vi "MT Generate PSK Symbol Map.vi"(0 "symbol values":i32[](array[numeric]), 11 "error in (no error)":errorcluster) -> (4 "symbol map":cdb[](array[numeric]) format="%.3f", 6 "bits per symbol":i32, 15 "error out":errorcluster)   [LabVIEW 2020, in "niDMT.lvlib"]
uses:
  <vilib>/addons/Modulation/niDMT.lvlib
  <vilib>/addons/Modulation/niAMT.lvlib
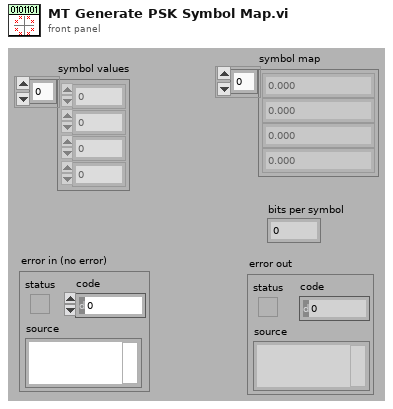
[diagram p1: front panel]
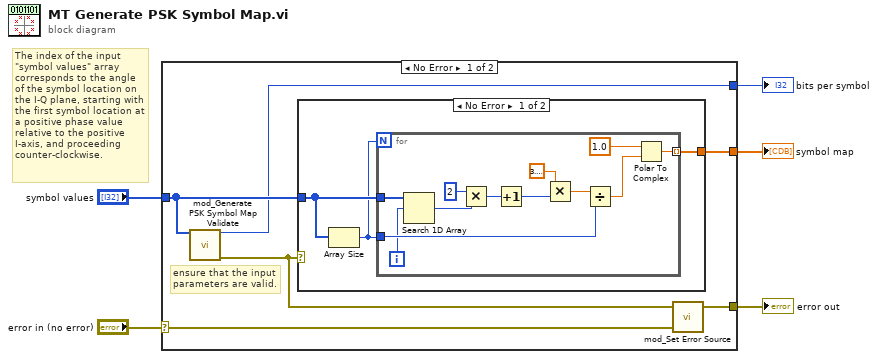
[diagram p0: block diagram]
diagram:
  # "The index of the input \"symbol values\" array corresponds to the angle of the symbol location on the I-Q plane, starting with the first symbol location at a positive phase value relative to the positive I-axis, and proceeding counter-clockwise."
  n1 = case shown="No Error" "error in (no error)" {
    selector: "error in (no error)" -> [w11 w27]
    tunnel: "symbol values" -> [w9 _]
    tunnel: [w10 w27] -> w4
    tunnel: [w8 _] -> w2
    tunnel: [w6 _] -> w1
    frame No Error {
      # "ensure that the input parameters are valid."
      n2 = call <vilib>:"mod_Generate PSK Symbol Map Validate.vi"("Symbol Map"=w9) -> ("bits per symbol"=w6:i32, "error out"=w7:errorcluster)  [unwired: 13 out]
      n3 = case shown="No Error" w7 {
        tunnel: w9 -> [w14 _]
        tunnel: [w13 _] -> w8
        frame No Error {
          n4 = Array Size(array=w14) -> (size(s)=w12:i32)
          n5 = for {
            N: w12 -> [_]
            tunnel: [w21] -> w13 mode=indexing
            tunnel: w14 -> [w19]
            tunnel: w12 -> [w20]
            i -> [w18]
            n6 = Search 1D Array(1D array=w19, element=w18) -> (index of element=w17:i32)  [unwired: 1 out]
            n7 = Multiply(x=2 ("y"), y=w17) -> (x*y=w23:i32)
            n8 = Increment(x=w23) -> (x+1=w15:i32)
            n9 = Multiply(x=3.141592653589793, y=w15) -> (x*y=w25:dbl)
            n10 = Divide(x=w25, y=w20) -> (x/y=w22:dbl)
            n11 = Polar To Complex(1:w22, 2:1.0) -> (0:w21:cdb)
          }
        }
        frame Error {
        }
      }
      n12 = call <vilib>:"mod_Set Error Source.vi"("initial error in (no error)"=w11, "final error in (no error)"=w7) -> ("error out"=w10:errorcluster)  [unwired: 3 out]
    }
    frame Error {
    }
  }
  "error out" <- w4
  "symbol map" <- w2
  "bits per symbol" <- w1
